vi "WaveformToAverageNPixels.vi"(0 "Waveform":waveform(dbl), 1 "N":i32) -> (2 "Pixels":dbl[](array[numeric]))   [LabVIEW 2009]
uses:
  <vilib>/Analysis/NI_AALBase.lvlib
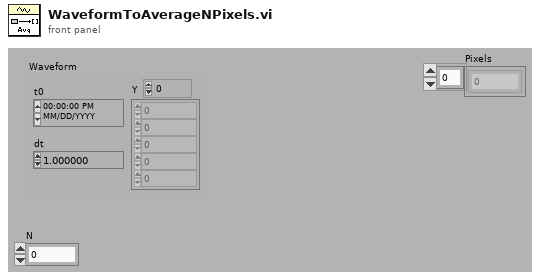
[diagram p1: front panel]
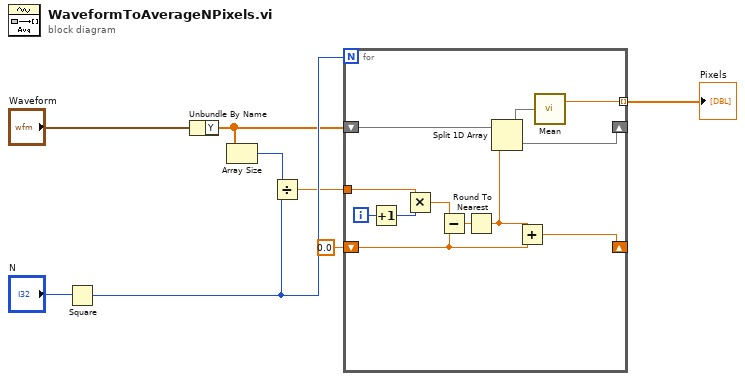
[diagram p0: block diagram]
diagram:
  n1 = Square(x="N") -> (x^2=w6:i32)
  n2 = Unbundle By Name("Waveform") -> ("Y"=w5:dbl[])
  n3 = Array Size(array=w5) -> (size(s)=w7:i32)
  n4 = Divide(x=w7, y=w6) -> (x/y=w4:dbl)
  n5 = for {
    N: w6 -> [_]
    shift-right: [w17] -> _
    shift-left: w5 -> [w18]
    tunnel: w4 -> [w20]
    shift-right: [w9] -> _
    shift-left: 0.0 -> [w10]
    tunnel: [w15] -> w2 mode=indexing
    i -> [w19]
    n6 = Increment(x=w19) -> (x+1=w13:i32)
    n7 = Multiply(x=w20, y=w13) -> (x*y=w12:dbl)
    n8 = Subtract(x=w12, y=w10) -> (x-y=w16:dbl)
    n9 = Round To Nearest(number=w16) -> (nearest integer value=w11:dbl)
    n10 = Split 1D Array(array=w18, index=w11) -> (first subarray=w14:dbl[], second subarray=w17:dbl[])
    n11 = Add(x=w11, y=w10) -> (x+y=w9:dbl)
    n12 = call <vilib>:"Mean.vi"("X"=w14) -> ("mean"=w15:dbl)  [unwired: 1 out]
  }
  "Pixels" <- w2
